vi "Nested Aliases.vi"(11 "jettl Queue Actor in":refnum<class "jettl Queue Actor.lvclass">) -> (2 "Nested Aliases":string[](array[string]))   [LabVIEW 2021, in "jettl.lvlib" / "jettl Queue Actor.lvlib" / "jettl Queue Actor.lvclass"]
uses:
  jettl Queue Actor.lvclass
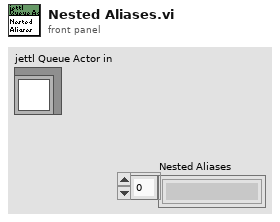
[diagram p1: front panel]
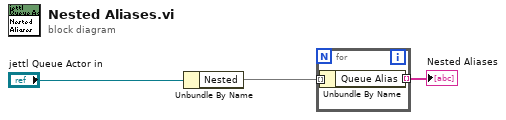
[diagram p0: block diagram]
diagram:
  n1 = Unbundle By Name("jettl Queue Actor in") -> ("Nested"=w2:map{string, refnum<data-value>})
  n2 = for {
    tunnel: [w4] -> w1 mode=indexing
    tunnel: w2 -> [w5] mode=indexing
    n3 = Unbundle By Name(w5) -> ("Queue Alias"=w4:string)
  }
  "Nested Aliases" <- w1
